vi "PV access control.vi"(7 "error in (no error)":errorcluster, 8 "PV access control - Cluster":T1={"Parameter"=enum."access request", "Parameter\nread only<->describe"=FALSE, "access locked\nreleased           locked "=TRUE, "access request"=2} {"access request" items=["--", "remote", "RS 485", "--", "PV.can", "--", "--", "--", "fieldbus"]}, 9 "Adress of unit":u16=1 max=999 step=1, 10 "VISA session":refnum<visa-resource-name>) -> (0 "error out":errorcluster, 2 "response (data)":string, 3 "dup VISA session":refnum<visa-resource-name>)   [LabVIEW 2016, in "Pfeiffer Vacuum.lvlib"]
doc: "There are 2 parameters available, only one of which can be enabled at a time. \n\naccess request (060)\naccess locked (061)\n\nNote: The controls right of this one will set the appropriate values for the selected parameter. Any settings for an parameter that is not selected will be ignored. If a value is out of range, it will be changed to either the upper or the lower limit of the range."
uses:
  Pfeiffer Vacuum.lvlib
  PV access control - Cluster.ctl
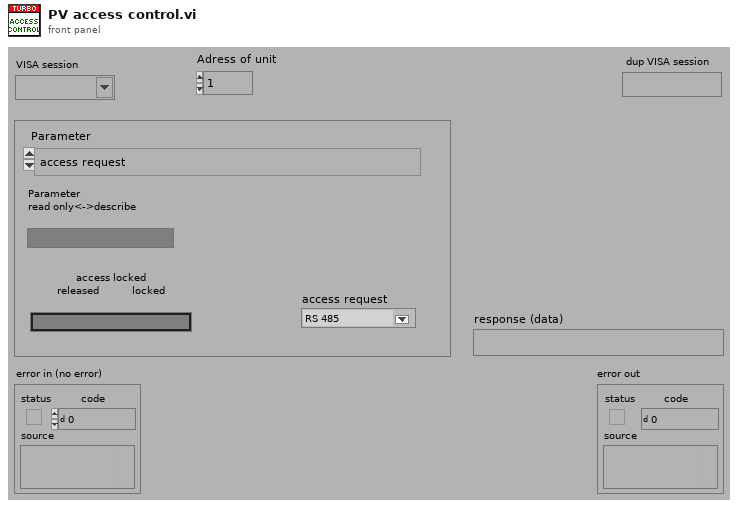
[diagram p1: front panel]
types:
  T1 = typedef "Pfeiffer Vacuum.lvlib/PV access control - Cluster.ctl" = cluster{"Parameter":enum16{"access request", "access locked"}, "Parameter\nread only<->describe":bool, "access locked\nreleased           locked ":bool, "access request":u16}
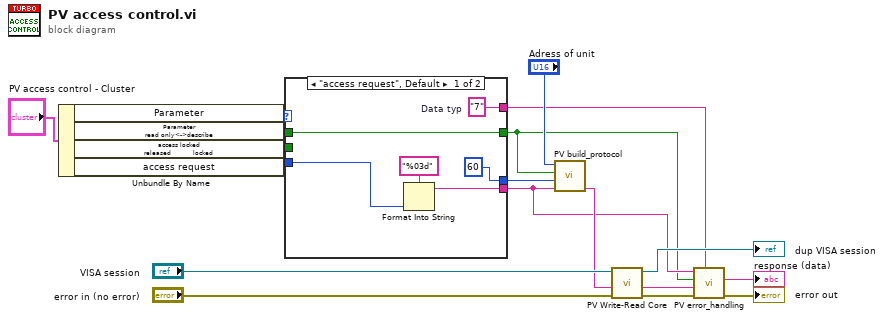
[diagram p0: block diagram]
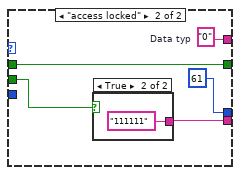
[diagram p2: hidden frame]
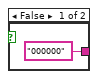
[diagram p3: hidden frame]
diagram:
  n1 = Unbundle By Name("PV access control - Cluster") -> ("Parameter"=w16:enum16{"access request", "access locked"}, "Parameter\nread only<->describe"=w15:bool, "access locked\nreleased           locked"=w14:bool, "access request"=w2:u16)
  n2 = case shown="\"access request\", Default" w16 {
    tunnel: [u16 60 ("Parameter-number") u16 61 ("Parameter-number")] -> w17
    tunnel: [w19 w25] -> w8
    tunnel: [w23 w28] -> w7
    tunnel: w15 -> [w23 w28]
    tunnel: w14 -> [_ w26]
    tunnel: [w22 w27] -> w9
    tunnel: w2 -> [w20 _]
    frame "access request", Default {
      w22 = "7"  # Data typ
      n3 = Format Into String(format string="%03d" ("Format-String"), w20) -> (resulting string=w19:string)  [unwired: 2 in, 1 out]
    }
    frame "access locked" {
      w27 = "0"  # Data typ
      n4 = case shown="True" w26 {
        tunnel: ["000000" ("Data") "111111" ("Data")] -> w25
        frame False {
        }
        frame True {
        }
      }
    }
  }
  n5 = call "PV build_protocol.vi"("Data"=w8, "Parameter-number"=w17, "parameter\nread<->describe"=w7, "Adress"="Adress of unit") -> ("output"=w11:string)  [unwired: 3 in]
  n6 = call "PV Write-Read Core.vi"("error in"="error in (no error)", "Write data in"=w11, "VISA session"="VISA session") -> ("error out"=w5:errorcluster, "response (data) out"=w6:string, "dup VISA session"=→"dup VISA session":refnum<visa-resource-name>)  [unwired: 2 in]
  n7 = call "PV error_handling.vi"("Data Typ in"=w9, "error in"=w5, "response (data) in"=w6, "Parameter\nread only<->describe"=w7, "data in"=w8) -> ("error out"=→"error out":errorcluster, "Data out"=→"response (data)":string)  [unwired: 4 in, 1 out]
